vi "Close.vi"(8 "error in (no error)":errorcluster, 11 "NiPxi6733 in":refnum<class "NiPxi6733.lvclass">) -> (0 "error out":errorcluster, 3 "NiPxi6733 out":refnum<class "NiPxi6733.lvclass">)   [LabVIEW 2014, in "FgenPlugins.lvlib" / "NiPxi6733.lvclass"]
uses:
  NiPxi6733.lvclass
  FgenPluginBaseClass/FgenPluginsBase.lvclass/FgenPluginsBase.ctl
  FgenPluginBaseClass/Accessors/Read Channels.vi
  FgenPluginBaseClass/Accessors/Write Channels.vi
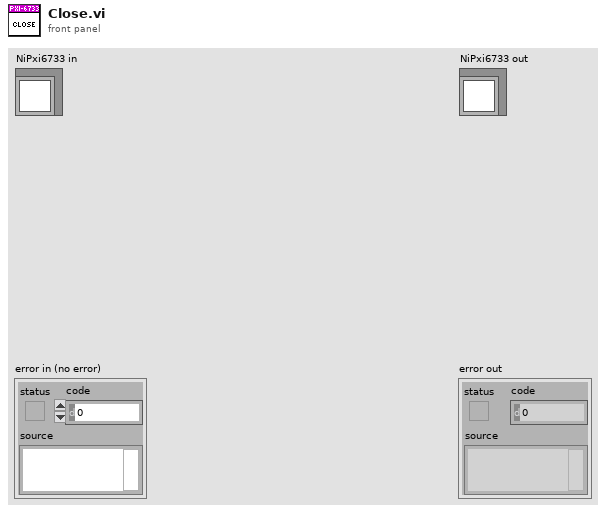
[diagram p1: front panel]
types:
  T1 = typedef "FgenPlugins.lvlib/Channel.ctl" = cluster{"Name":string, "Enabled":bool, "Operation":enum16{"Continuous", "Burst"}, "Impedance (50)":dbl, "Handle":string, "Connected":bool, "Mode (Function)":enum16{"Function", "Arbitrary", "Sequence"}}
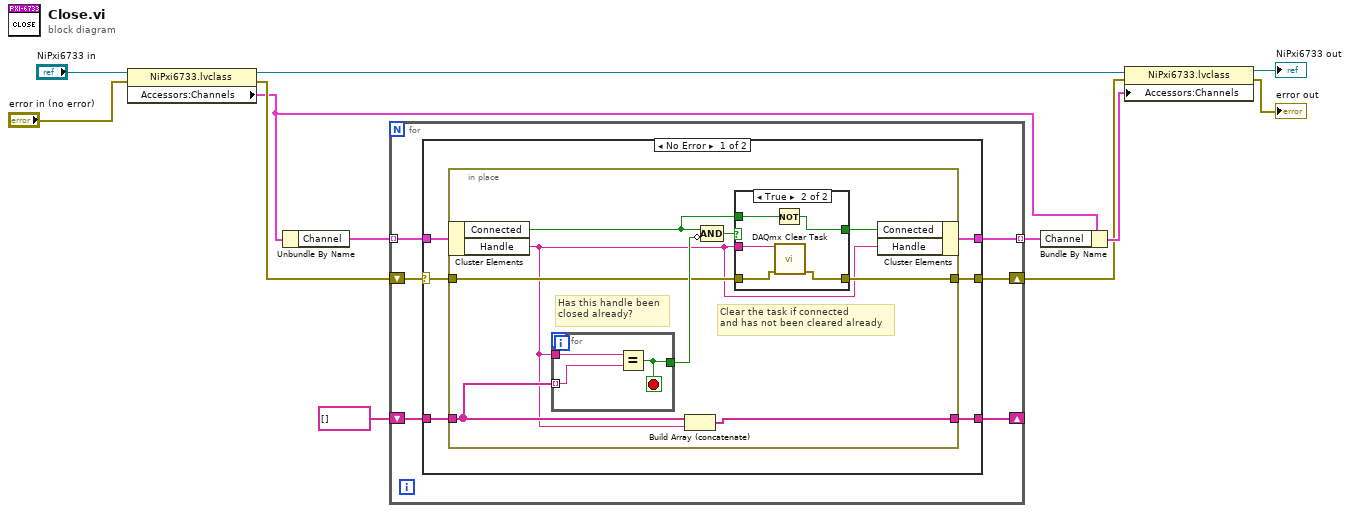
[diagram p0: block diagram]
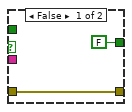
[diagram p2: hidden frame]
diagram:
  n1 = property class="NiPxi6733.lvclass"(reference="NiPxi6733 in", error in="error in (no error)") -> (reference out=w4:refnum<class "NiPxi6733.lvclass">, error out=w10:errorcluster, "Accessors:Channels"=w6:cluster{"Count":u16, "Channel":T1[]})
  n2 = Unbundle By Name(w6) -> ("Channel"=w9:T1[])
  n3 = for {
    shift-right: [w15] -> w1
    shift-left: w10 -> [w18]
    tunnel: w9 -> [w17] mode=indexing
    shift-right: [w13] -> _
    shift-left: string[] [] -> [w16]
    tunnel: [w14] -> w7 mode=indexing
    n4 = case shown="No Error" w18 {
      selector: w18 -> [w22 w46]
      tunnel: w17 -> [w24 w45]
      tunnel: w16 -> [w23 w44]
      tunnel: [w21 w46] -> w15
      tunnel: [w20 w45] -> w14
      tunnel: [w19 w44] -> w13
      frame No Error {
        n5 = in-place {
          in-place-border: w23 -> [w27]
          in-place-border: w22 -> [w31]
          in-place-border: [w30] -> w21
          in-place-border: [w25] -> w19
          # "Clear the task if connected\nand has not been cleared already"
          # "Has this handle been\nclosed already?"
          n6 = in-place-cluster #1(w24) -> ("Connected"=w29:bool, "Handle"=w26:string)
          n7 = for {
            tunnel: w27 -> [w41] mode=indexing
            tunnel: w26 -> [w43]
            tunnel: [w42] -> w33
            stop <- w42 stop-if-true
            n8 = Equal?(x=w43, y=w41) -> (x = y?=w42:bool)
          }
          n9 = Build Array (concatenate)(w27, w26) -> (w25:string[])
          n10 = Compound Arithmetic op=AND(w29, invert w33) -> (w32:bool)
          n11 = case shown="True" w32 {
            tunnel: w26 -> [_ w40]
            tunnel: w31 -> [w34 w39]
            tunnel: [w34 w38] -> w30
            tunnel: w29 -> [_ w37]
            tunnel: [FALSE w36] -> w28
            frame False {
            }
            frame True {
              n12 = Not(x=w37) -> (.not. x?=w36:bool)
              n13 = call <vilib>:"DAQmx Clear Task.vi"("task in"=w40, "error in"=w39) -> ("error out"=w38:errorcluster)  [unwired: 13 in]
            }
          }
          n14 = in-place-cluster #1("Connected"=w28, "Handle"=w26) -> (w20:T1)
        }
      }
      frame Error {
      }
    }
  }
  n15 = Bundle By Name(cluster=w6, "Channel"=w7) -> (w5:cluster{"Count":u16, "Channel":T1[]})
  n16 = property class="NiPxi6733.lvclass"(reference=w4, error in=w1, "Accessors:Channels"=w5) -> (reference out=→"NiPxi6733 out":refnum<class "NiPxi6733.lvclass">, error out=→"error out":errorcluster)
